vi "sortowanie po kącie.vi"(2 "error in (no error)":errorcluster, 3 "unsorted array":dbl[][](array[numeric])) -> (0 "error out":errorcluster, 1 "sorted array":dbl[][](array[numeric]))   [LabVIEW 2016]
uses:
  09846a0b-ee68-4165-ab15-71064aba3c77.vi
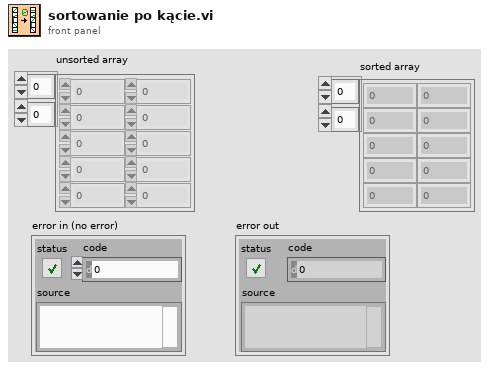
[diagram p1: front panel]
types:
  T1 = cluster{"Numeric":dbl, "Numeric":dbl, "Numeric":dbl}
  T2 = cluster{"Numeric":dbl, "Numeric":dbl, "Numeric":dbl}[]
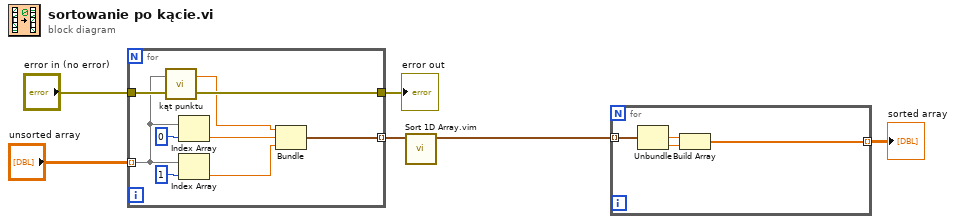
[diagram p0: block diagram]
diagram:
  n1 = for {
    tunnel: "unsorted array" -> [w8] mode=indexing
    tunnel: [w13] -> w3 mode=indexing
    tunnel: "error in (no error)" -> [w12]
    tunnel: [w11] -> w4
    n2 = call "kąt punktu.vi"("error in (no error)"=w12, "Pkt"=w8) -> ("error out"=w11:errorcluster, "Numeric"=w7:dbl)
    n3 = Index Array(array=w8, index=0) -> (element=w10:dbl)
    n4 = Index Array(array=w8, index=1) -> (element=w9:dbl)
    n5 = Bundle("Numeric"=w7, "Numeric"=w10, "Numeric"=w9) -> (w13:T1)  [unwired: 1 in]
  }
  "error out" <- w4
  n6 = call "Sort 1D Array.vim"("unsorted array"=w3) -> ("sorted array"=w2:T2)  [unwired: 10 in]
  n7 = for {
    tunnel: w2 -> [w19] mode=indexing
    tunnel: [w16] -> w1 mode=indexing
    n8 = Unbundle(w19) -> ("Numeric"=w18:dbl, "Numeric"=w17:dbl)  [unwired: 1 out]
    n9 = Build Array(w18, w17) -> (w16:dbl[])
  }
  "sorted array" <- w1
